vi "Read.vi"(6 "Qbus in":refnum<class "Qbus.lvclass">, 8 "error in (no error)":errorcluster, 10 "channel":T1, 11 "reference":refnum<class "Modbus Master.lvclass">) -> (0 "error out":errorcluster, 4 "read error":errorcluster)   [LabVIEW 2017, in "ModbusMaster.lvlib"]
uses:
  <vilib>/addons/InsightCM/Devices/Shared/Common/ModbusMaster/ModbusMaster.lvlib
  <vilib>/addons/InsightCM/Devices/Shared/Common/ModbusMaster/controls/ModbusChannel.ctl
  <vilib>/addons/InsightCM/Devices/Shared/Common/ModbusMaster/controls/RegisterType.ctl
  <vilib>/Modbus/master/Modbus Master.lvclass
  <vilib>/addons/Qbus/Qbus.lvclass
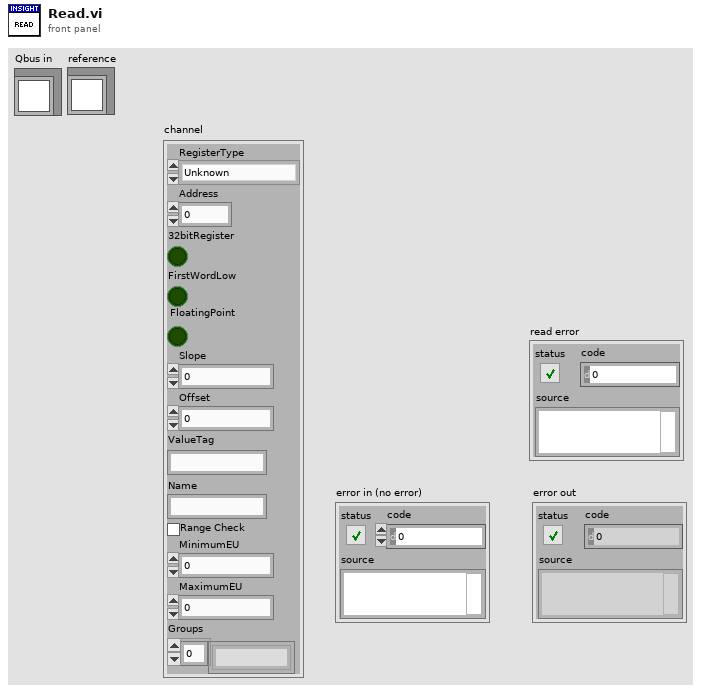
[diagram p1: front panel]
types:
  T1 = typedef "ModbusMaster.lvlib/ModbusChannel.ctl" = cluster{"RegisterType":T2, "Address":i32, "32bitRegister":bool, "FirstWordLow":bool, "FloatingPoint":bool, "Slope":dbl, "Offset":dbl, "ValueTag":string, "Name":string, "Range Check":bool, "MinimumEU":dbl, "MaximumEU":dbl, "Groups":string[]}
  T2 = typedef "ModbusMaster.lvlib/RegisterType.ctl" = enum16{"Unknown", "Coil", "Discrete Input", "Holding Register", "Input Register"}
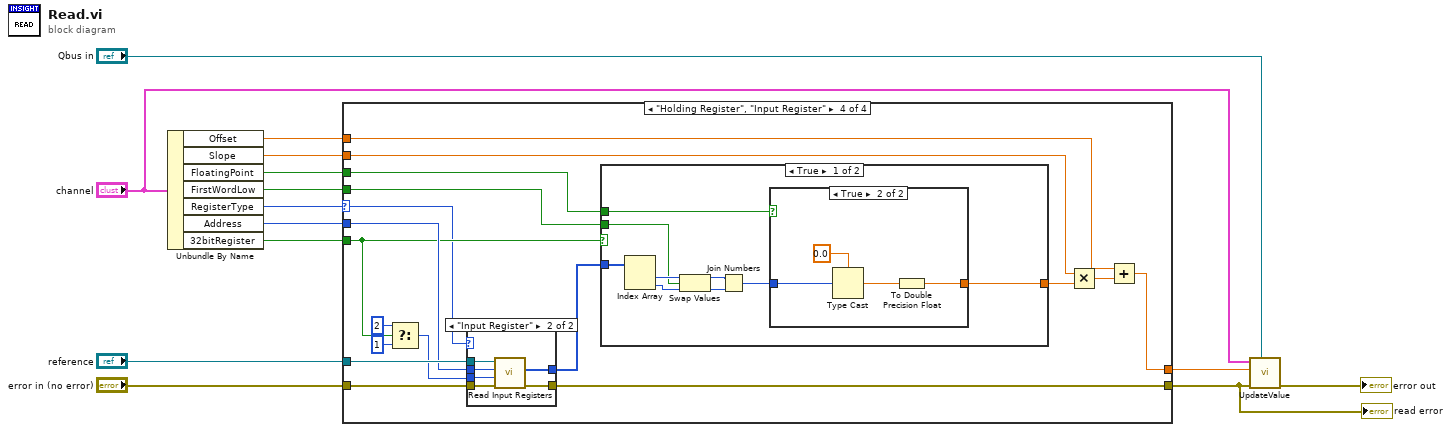
[diagram p0: block diagram]
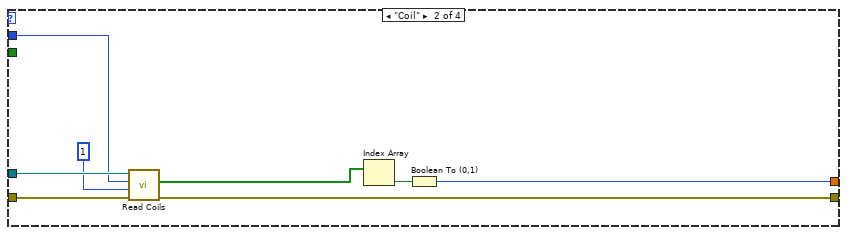
[diagram p3: hidden frame]
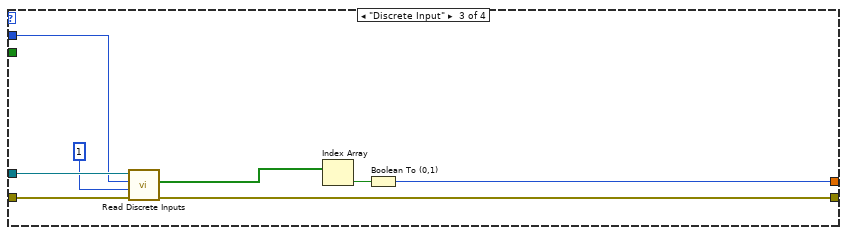
[diagram p4: hidden frame]
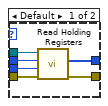
[diagram p5: hidden frame]
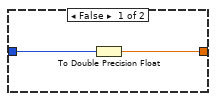
[diagram p6: hidden frame]
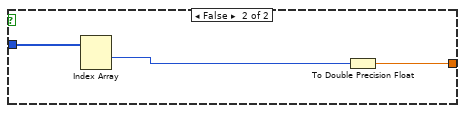
[diagram p7: hidden frame]
diagram:
  n1 = Unbundle By Name("channel") -> ("Offset"=w6:dbl, "Slope"=w7:dbl, "FloatingPoint"=w8:bool, "FirstWordLow"=w1:bool, "RegisterType"=w14:T2, "Address"=w12:i32, "32bitRegister"=w9:bool)
  n2 = case shown="\"Holding Register\", \"Input Register\"" w14 {
    selector: w14 -> [_ _ _ w39]
    tunnel: "error in (no error)" -> [w15 w23 w27 w45]
    tunnel: "reference" -> [_ w22 w30 w48]
    tunnel: w12 -> [_ w21 w26 w47]
    tunnel: [w15 w17 w28 w46] -> w5
    tunnel: [_ w16 w24 w34] -> w10
    tunnel: w9 -> [_ _ _ w41]
    tunnel: w8 -> [_ _ _ w38]
    tunnel: w7 -> [_ _ _ w37]
    tunnel: w6 -> [_ _ _ w33]
    tunnel: w1 -> [_ _ _ w32]
    frame "Unknown" {
    }
    frame "Coil" {
      n3 = call-dynamic "Read Coils.vi"("error in (no error)"=w23, "number of coils"=u16 1, "starting address"=w21, "Modbus master in"=w22) -> ("error out"=w17:errorcluster, "coil values"=w19:bool[])  [unwired: 5 in, 1 out]
      n4 = Index Array(array=w19) -> (element=w18:bool)  [unwired: 1 in]
      n5 = Boolean To (0,1)(Boolean=w18) -> (0, 1=w16:i16)
    }
    frame "Discrete Input" {
      n6 = call-dynamic "Read Discrete Inputs.vi"("error in (no error)"=w27, "number of discrete inputs"=u16 1 ("number of coils"), "starting address"=w26, "Modbus master in"=w30) -> ("error out"=w28:errorcluster, "discrete input values"=w29:bool[])  [unwired: 5 in, 1 out]
      n7 = Index Array(array=w29) -> (element=w31:bool)  [unwired: 1 in]
      n8 = Boolean To (0,1)(Boolean=w31) -> (0, 1=w24:i16)
    }
    frame "Holding Register", "Input Register" {
      n9 = Select(t=u16 2 ("number of coils"), s=w41, f=u16 1 ("number of coils")) -> (s? t:f=w42:u16)
      n10 = case shown="\"Input Register\"" w39 {
        tunnel: w48 -> [w54 w60]
        tunnel: w47 -> [w53 w57]
        tunnel: [w52 w55] -> w46
        tunnel: w45 -> [w51 w59]
        tunnel: w42 -> [w50 w58]
        tunnel: [w49 w56] -> w40
        frame Default {
          n11 = call-dynamic "Read Holding Registers.vi"("error in (no error)"=w51, "number of holding registers"=w50, "starting address"=w53, "Modbus master in"=w54) -> ("error out"=w52:errorcluster, "register values"=w49:u16[])  [unwired: 5 in, 1 out]
        }
        frame "Input Register" {
          n12 = call-dynamic "Read Input Registers.vi"("error in (no error)"=w59, "number of input registers"=w58, "starting address"=w57, "Modbus master in"=w60) -> ("error out"=w55:errorcluster, "register values"=w56:u16[])  [unwired: 5 in, 1 out]
        }
      }
      n13 = case shown="True" w41 {
        tunnel: w40 -> [w69 w78]
        tunnel: w38 -> [w63 _]
        tunnel: [w61 w76] -> w36
        tunnel: w32 -> [w64 _]
        frame True {
          n14 = Index Array(array=w69) -> (element #1=w68:u16, element #2=w67:u16)  [unwired: 2 in]
          n15 = Swap Values(12:w68, 13:w64, 14:w67) -> (1:w66:u16, 3:w65:u16)
          n16 = Join Numbers(hi=w66, lo=w65) -> ((hi.lo)=w62:u32)
          n17 = case shown="True" w63 {
            tunnel: w62 -> [w71 w75]
            tunnel: [w70 w72] -> w61
            frame False {
              n18 = To Double Precision Float(number=w71) -> (double precision float=w70:dbl)
            }
            frame True {
              n19 = Type Cast(type=sgl 0.0, x=w75) -> (*(type *) &x=w73:sgl)
              n20 = To Double Precision Float(number=w73) -> (double precision float=w72:dbl)
            }
          }
        }
        frame False {
          n21 = Index Array(array=w78) -> (element #1=w77:u16)  [unwired: 2 in, 1 out]
          n22 = To Double Precision Float(number=w77) -> (double precision float=w76:dbl)
        }
      }
      n23 = Multiply(x=w37, y=w36) -> (x*y=w35:dbl)
      n24 = Add(x=w33, y=w35) -> (x+y=w34:dbl)
    }
  }
  "read error" <- w5
  n25 = call <vilib>:"UpdateValue.vi"("Qbus in"="Qbus in", "error in (no error)"=w5, "Numeric"=w10, "channel"="channel") -> ("error out"=→"error out":errorcluster)  [unwired: 7 in]
